vi "Set Edges.vi"(11 "Plant Regions in":map{T1, u32}[](array[numeric])) -> (3 "Plant Regions out":map{T1, u32}[](array[numeric]))   [LabVIEW 2024]
uses:
  Utility/Universal Utility/TypeDefs_Utility/Cluster_Row-Column.ctl
  Utility/Universal Utility/TypeDefs_Utility/ENUM_4 Directions U-D-L-R.ctl
  <vilib>/Utility/miscctls.llb/LVMapReplaceAction.ctl
  9ec40043-fd1c-4aa8-aa2f-c598280360ae.vi
  9ec40043-fd1c-4aa8-aa2f-c598280360ae.vi/0a5f5d0f-6921-449f-9499-5f6c7f3eae0e.vi
  9ec40043-fd1c-4aa8-aa2f-c598280360ae.vi/2f57c213-34d0-4fb8-93c4-9da21d141025.vi
  <vilib>/Utility/error.llb/Trim Whitespace.vi
  <vilib>/Utility/error.llb/Trim Whitespace One-Sided.vi
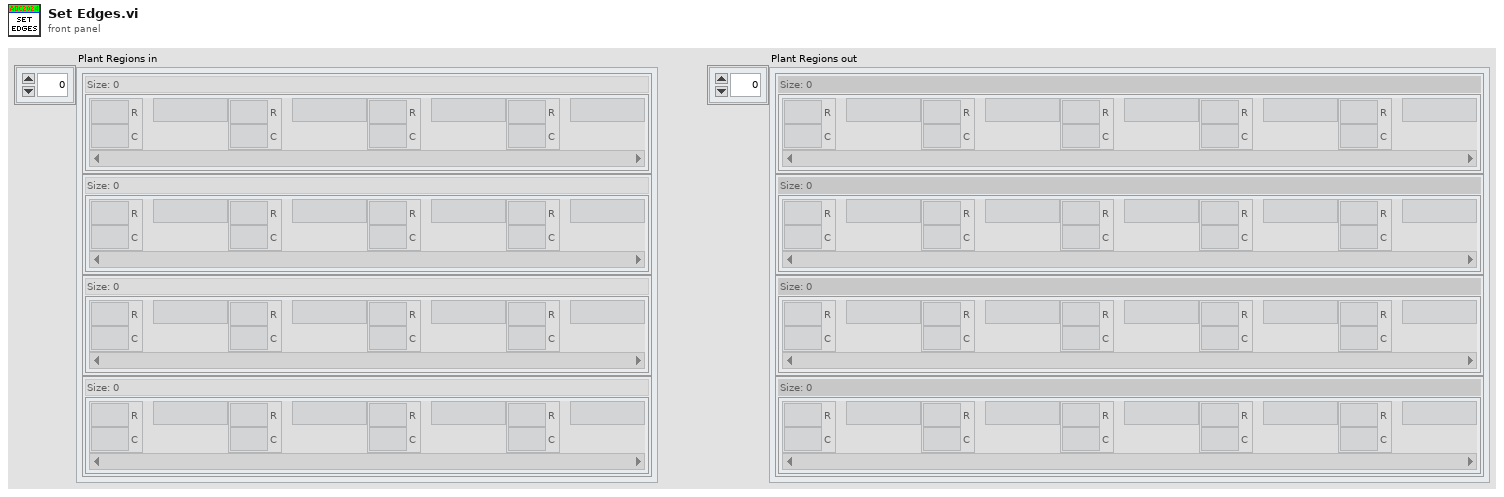
[diagram p1: front panel]
types:
  T1 = typedef "Cluster_Row-Column.ctl" = cluster{"R":i32, "C":i32}
  T2 = typedef "ENUM_4 Directions U-D-L-R.ctl" = enum16{"Up;-1,0", "Right;0,1", "Down;1,0", "Left;0,-1"}
  T3 = typedef "LVMapReplaceAction.ctl" = enum32{"Modify Entry only if found", "Add or Modify Entry", "Delete Entry"}
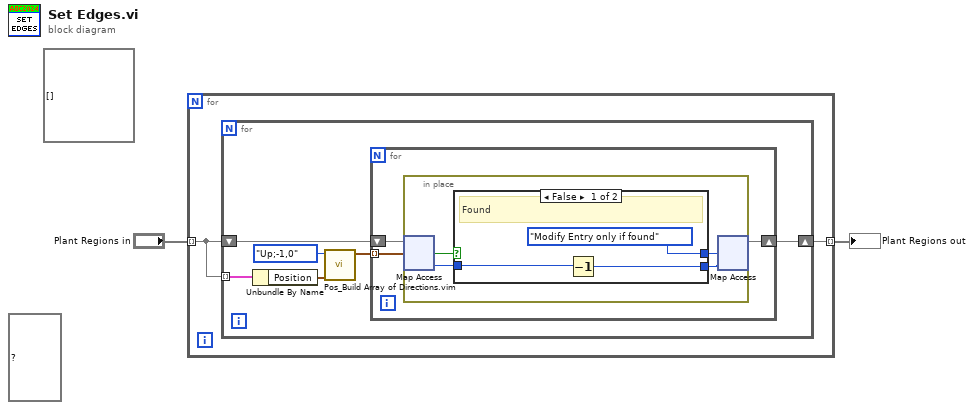
[diagram p0: block diagram]
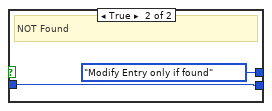
[diagram p2: hidden frame]
diagram:
  (unwired) map{T1, u32} {} ("Perimeter")
  (unwired) map{T1, u32}[] [] ("Plant Regions in")
  n1 = for {
    tunnel: "Plant Regions in" -> [w4] mode=indexing
    tunnel: [w3] -> w1 mode=indexing
    n2 = for {
      tunnel: w4 -> [w10] mode=indexing
      shift-right: [w7] -> w3
      shift-left: w4 -> [w8]
      n3 = Unbundle By Name(w10) -> ("Position"=w6:T1)
      n4 = call "Pos_Build Array of Directions.vim"("Positon"=w6, "Direction"=ENUM_4_Directions_U-D-L-R."Up;-1,0") -> ("Direction Positions Out"=w5:T1[])  [unwired: 9 in]
      n5 = for {
        tunnel: w5 -> [w12] mode=indexing
        shift-right: [w11] -> w7
        shift-left: w8 -> [w13]
        n6 = in-place {
          n7 = in-place-map #1(w13, w12) -> (w17:u32, w14:bool)  [unwired: 1 in]
          n8 = case shown="False" w14 {
            tunnel: w17 -> [w20 w22]
            tunnel: [w19 w22] -> w16
            tunnel: [LVMapReplaceAction."Modify Entry only if found" ("action") LVMapReplaceAction."Modify Entry only if found" ("action")] -> w15
            frame False {
              # "Found"
              n9 = Decrement(x=w20) -> (x-1=w19:u32)
            }
            frame True {
              # "NOT Found"
            }
          }
          n10 = in-place-map #1(w16, w15) -> (w11:map{T1, u32})  [unwired: 2 out]
        }
      }
    }
  }
  "Plant Regions out" <- w1
